vi "VS_UpdateParamFromFile.vi"(0 "Engine Reference(in)":refnum<k7>, 1 "Condition Run?":bool, 5 "Sequence File Ref(in)":refnum<k7>, 7 "VeriStand version info":T1, 9 "Parameter Value array":string[][](array[string]), 11 "error in":errorcluster, 12 "Step Group":i32(ring) items=["StepGroup_Setup", "StepGroup_Main", "StepGroup_Cleanup"], 13 "Step Index":i32, 14 "Requirement":string) -> (4 "Engine reference(out)":refnum<k7>, 6 "Sequence File Ref(out)":refnum<k7>, 8 "VeriStand version info (out)":T1, 15 "error out":errorcluster)   [LabVIEW 2010]
doc: "This VI creates a VeriStand step in TestStand to update parameters through an .m file"
uses:
  Ctls/dotNetAssemblyInfo.ctl
  Ctls/VSModuleTokens.ctl
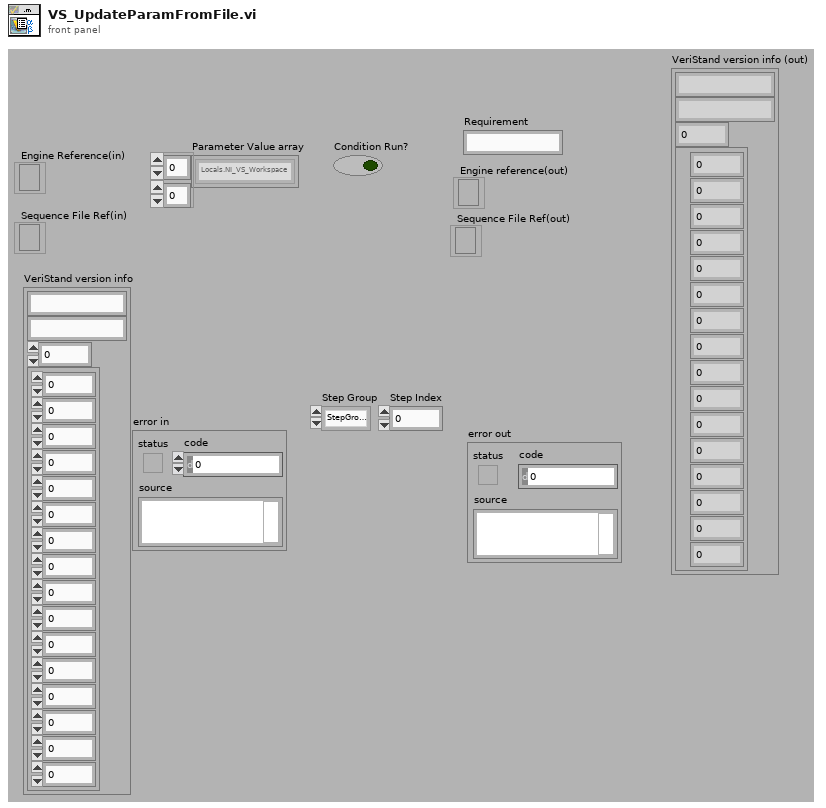
[diagram p1: front panel]
types:
  T1 = typedef "dotNetAssemblyInfo.ctl" = cluster{"VeriStand.exe Path":string, "Assembly":string, "Constructor Token":i32, "Module Token":T2}
  T2 = typedef "VSModuleTokens.ctl" = cluster{"GetIWorkspaceToken":i32, "GetIStimulusToken":i32, "GetIModelManagerToken":i32, "GetIProjectToken":i32, "RunProjectToken":i32, "CloseProjectToken":i32, "RunWorkspaceToken":i32, "StopWorkspaceToken":i32, "SetSingleChannelToken":i32, "SetMultipleParametersToken":i32, "RunStimulusToken":i32, "GetStimulusStateToken":i32, "Open WorkspaceToken":i32, "DeployToken":i32, "UndeployToken":i32, "QuitToken":i32}
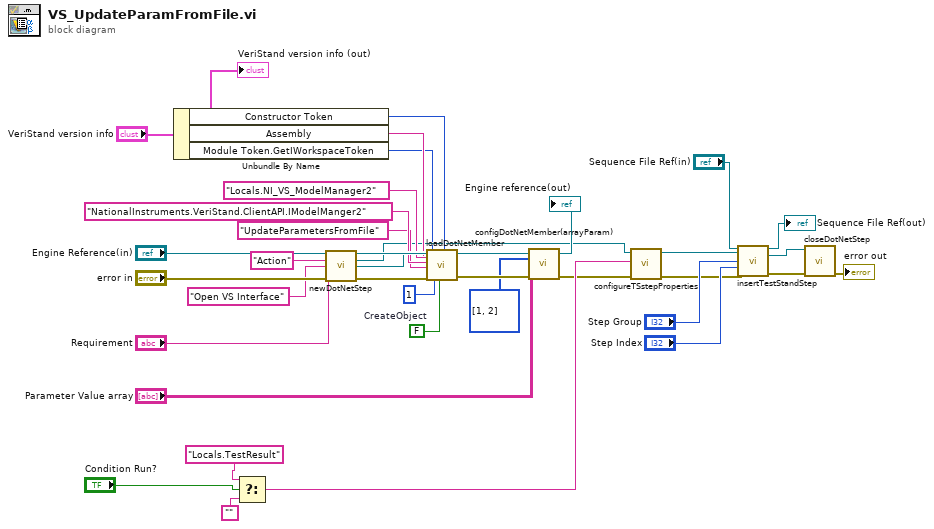
[diagram p0: block diagram]
diagram:
  w20 = FALSE  # CreateObject
  n1 = Unbundle By Name("VeriStand version info") -> ("Constructor Token"=w14:i32, "Assembly"=w15:string, "Module Token.GetIWorkspaceToken"=w3:i32)
  n2 = Select(t="Locals.TestResult", s="Condition Run?", f="") -> (s? t:f=w6:string)
  n3 = call "newDotNetStep.vi"("Engine reference"="Engine Reference(in)", "stepType"="Action", "Step Name"="Open VS Interface", "Requirement"="Requirement", "error in"="error in") -> ("Engine reference(out)"=→"Engine reference(out)":refnum<k7>, "NewStep (out)"=w8:refnum<k7>, "dotNetModule(out)"=w24:refnum<k7>, "error out"=w36:errorcluster)  [unwired: 7 in]
  n4 = call "loadDotNetMember.vi"("dotNetModule"=w24, "Strong Assembly path"=w15, "ClassName"="NationalInstruments.VeriStand.ClientAPI.IModelManger2", "MemberName"="UpdateParametersFromFile", "Member token"=w3, "error in(no error)"=w36, "ClassReference"="Locals.NI_VS_ModelManager2", "Call Member?"=1 ("Call Memeber?"), "CreateObject"=w20, "Constructor Token"=w14) -> ("dotNetModule(out)"=w19:refnum<k7>, "error out"=w18:errorcluster)  [unwired: 8 in]
  n5 = call "configDotNetMember(arrayParam).vi"("dotNetModule"=w19, "Index array"=i32[] [1, 2], "Parameter Value array"="Parameter Value array", "error in (no error)"=w18) -> ("error out"=w5:errorcluster)  [unwired: 11 in]
  n6 = call "configureTSstepProperties.vi"("error in"=w5, "Precondition"=w6, "NewStep (in)"=w8) -> ("error out"=w4:errorcluster, "NewStep (out)"=w7:refnum<k7>)  [unwired: 7 in]
  n7 = call "insertTestStandStep.vi"("Sequence File Ref"="Sequence File Ref(in)", "Step to insert"=w7, "Step Group"="Step Group", "index"="Step Index", "error out"=w4) -> ("Sequence File Ref(out)"=→"Sequence File Ref(out)":refnum<k7>, "Step to insert (out)"=w35:refnum<k7>, "error out"=w33:errorcluster)  [unwired: 8 in]
  n8 = call "closeDotNetStep.vi"("error in"=w33, "NewStep"=w35) -> ("error out"=→"error out":errorcluster)  [unwired: 9 in]
  "VeriStand version info (out)" <- "VeriStand version info"
